vi "SubCalEdgePoint.vi"(0 "Image dup":T1, 1 "Mid Point Top World X":sgl, 2 "Mid Point Top World Y":sgl, 7 "Mid Point":dbl[](array[numeric]), 9 "Left Point":dbl[](array[numeric]), 11 "Right Point":dbl[](array[numeric]), 12 "Mid Point Base World X":sgl, 13 "Mid Point Base World Y":sgl) -> (4 "Edge Lefe Side":cluster{cluster{"Xln":dbl, "Yln":dbl}}[][](array[cluster]), 15 "Edge Right Side":cluster{cluster{"Xrn":dbl, "Yrn":dbl}}[][](array[cluster]))   [LabVIEW 2015]
uses:
  <vilib>/vision/Image Controls.llb/IMAQ Image.ctl
  <vilib>/vision/NI_Vision_Development_Module.lvlib
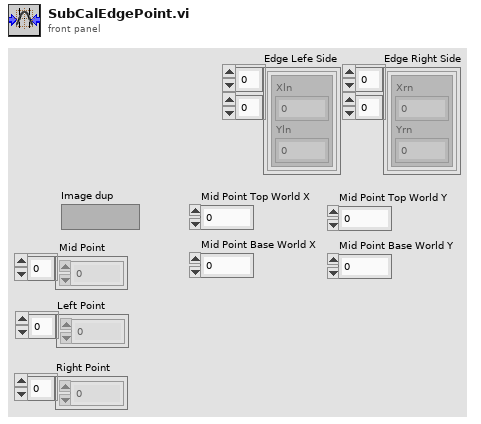
[diagram p1: front panel]
types:
  T1 = typedef "IMAQ Image.ctl" = refnum<image>
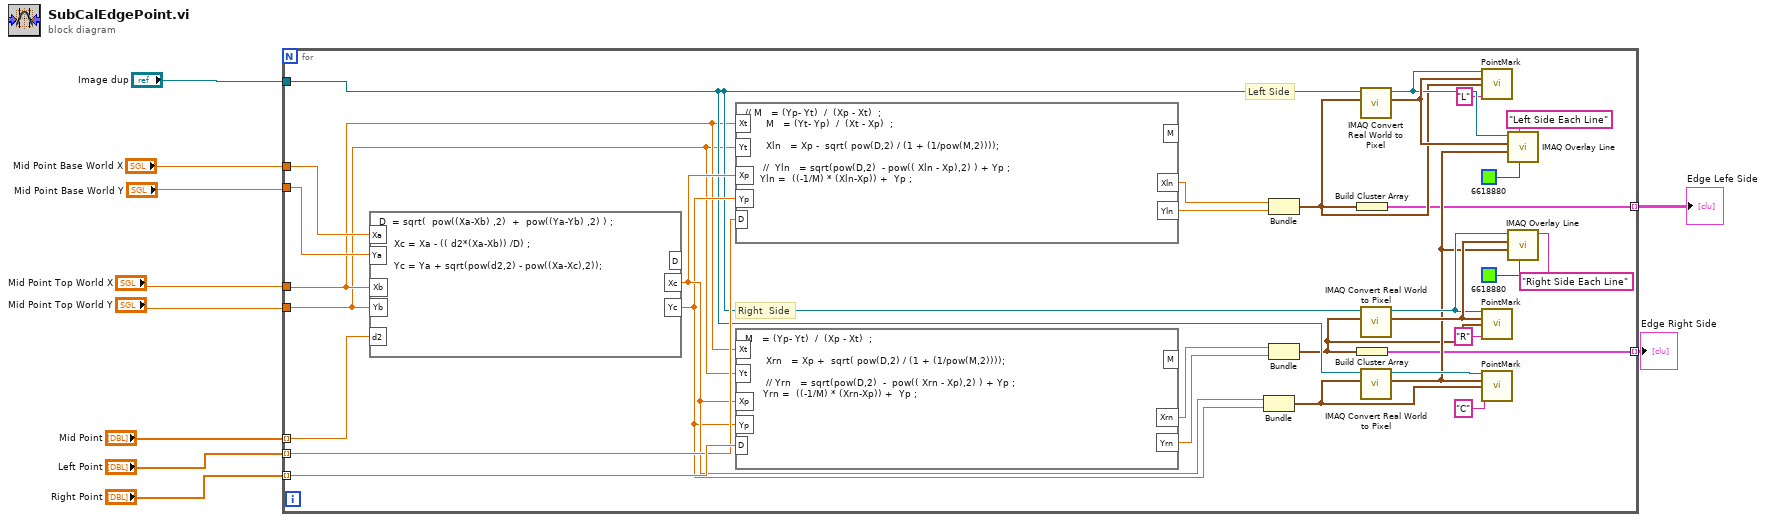
[diagram p0: block diagram]
diagram:
  n1 = for {
    tunnel: "Mid Point" -> [w41] mode=indexing
    tunnel: "Mid Point Top World Y" -> [w22]
    tunnel: "Mid Point Top World X" -> [w23]
    tunnel: "Mid Point Base World X" -> [w25]
    tunnel: "Mid Point Base World Y" -> [w24]
    tunnel: "Image dup" -> [w33]
    tunnel: "Left Point" -> [w37] mode=indexing
    tunnel: "Right Point" -> [w38] mode=indexing
    tunnel: [w16] -> w2 mode=indexing
    tunnel: [w14] -> w1 mode=indexing
    # "Left Side"
    # "Right  Side"
    n2 = formula code="D  = sqrt(  pow((Xa-Xb) ,2)  +  pow((Ya-Yb) ,2) ) ;\n\n     Xc = Xa - (( d2*(Xa-Xb)) /D) ;  \n \n     Yc = Ya + sqrt(pow(d2,2) - pow((Xa-Xc),2));"("Xa"=w25, "Xb"=w23, "Ya"=w24, "Yb"=w22, "d2"=w41) -> ("Xc"=w36:dbl, "Yc"=w35:dbl)  [unwired: 1 out]
    n3 = formula code="// M   = (Yp- Yt)  /  (Xp - Xt)  ; \n       M   = (Yt- Yp)  /  (Xt - Xp)  ; \n\n       Xln   = Xp -  sqrt( pow(D,2) / (1 + (1/pow(M,2)))); \n\n      //  Yln   = sqrt(pow(D,2)  - pow(( Xln - Xp),2) ) + Yp ; \n     Yln =  ((-1/M) * (Xln-Xp)) +  Yp ;"("Xt"=w23, "Yt"=w22, "Xp"=w36, "Yp"=w35, "D"=w37) -> ("Xln"=w21:dbl, "Yln"=w20:dbl)  [unwired: 1 out]
    n4 = formula code="M   = (Yp- Yt)  /  (Xp - Xt)  ; \n\n       Xrn   = Xp +  sqrt( pow(D,2) / (1 + (1/pow(M,2)))); \n\n       // Yrn   = sqrt(pow(D,2)  -  pow(( Xrn - Xp),2) ) + Yp ; \n      Yrn =  ((-1/M) * (Xrn-Xp)) +  Yp ;"("Xt"=w23, "Yt"=w22, "Xp"=w36, "Yp"=w35, "D"=w38) -> ("Xrn"=w19:dbl, "Yrn"=w18:dbl)  [unwired: 1 out]
    n5 = Bundle("Xc"=w36, "Yc"=w35) -> (w39:cluster{"Xc":dbl, "Yc":dbl})  [unwired: 1 in]
    n6 = Bundle("Xln"=w21, "Yln"=w20) -> (w17:cluster{"Xln":dbl, "Yln":dbl})  [unwired: 1 in]
    n7 = Bundle("Xrn"=w19, "Yrn"=w18) -> (w15:cluster{"Xrn":dbl, "Yrn":dbl})  [unwired: 1 in]
    n8 = Build Cluster Array(w17) -> (w16:cluster{cluster{"Xln":dbl, "Yln":dbl}}[])
    n9 = Build Cluster Array(w15) -> (w14:cluster{cluster{"Xrn":dbl, "Yrn":dbl}}[])
    n10 = call "IMAQ Convert Real World to Pixel"("Real World Coordinates"=w17, "Calibrated Image"=w33) -> ("Pixel Coordinates"=w29:cluster{"X":sgl, "Y":sgl}, "Calibrated Image (duplicate)"=w28:T1)  [unwired: 4 in, 4 out]
    n11 = call "IMAQ Convert Real World to Pixel"("Real World Coordinates"=w15, "Calibrated Image"=w33) -> ("Pixel Coordinates"=w32:cluster{"X":sgl, "Y":sgl}, "Calibrated Image (duplicate)"=w31:T1)  [unwired: 4 in, 4 out]
    n12 = call "IMAQ Convert Real World to Pixel"("Real World Coordinates"=w39, "Calibrated Image"=w33) -> ("Pixel Coordinates"=w27:cluster{"X":sgl, "Y":sgl}, "Calibrated Image (duplicate)"=w42:T1)  [unwired: 4 in, 4 out]
    n13 = call "PointMark.vi"("Refnum in"=w28, "Position Pixel"=w29, "Position World"=w17, "String"="L") -> ()  [unwired: 12 in]
    n14 = call "PointMark.vi"("Refnum in"=w31, "Position Pixel"=w32, "Position World"=w15, "String"="R") -> ()  [unwired: 12 in]
    n15 = call "PointMark.vi"("Refnum in"=w42, "Position Pixel"=w27, "Position World"=w39, "String"="C") -> ()  [unwired: 12 in]
    n16 = call "IMAQ Overlay Line"("Color"=u32 6618880, "Group"="Left Side Each Line", "End Point"=w27, "Start Point"=w29, "Image"=w28) -> ()  [unwired: 5 in, 2 out]
    n17 = call "IMAQ Overlay Line"("Color"=u32 6618880, "Group"="Right Side Each Line", "End Point"=w27, "Start Point"=w32, "Image"=w31) -> ()  [unwired: 5 in, 2 out]
  }
  "Edge Lefe Side" <- w2
  "Edge Right Side" <- w1
